vi "MLClassification.vi"(9 "with labels?":bool, 10 "Frame data":string[](array[string]), 11 "model file (JSON)":path) -> (0 "error out":errorcluster, 1 "metrics":T1, 2 "predicted result":i32[][](graph), 3 "feature trend":dbl[][](graph), 5 "Detected hand sign":i32)   [LabVIEW 2017, in "MachineLearning.lvlib"]
doc: "Demonstrates how to deploy a trained classification model to classify test data."
uses:
  MachineLearning.lvlib
  TypeDefs/Label Setting.ctl
  <vilib>/addons/AML/Common/Classes/AML Analytics Model.lvclass/AML Analytics Model.ctl
  <vilib>/addons/AML/Common/Classes/aml_Read Feature Manipulation Model Type.vi
  <vilib>/addons/AML/Data/Load Testing Data (2D Array).vi
  <vilib>/addons/AML/Analytics and Machine Learning.lvlib
  <vilib>/addons/AML/Common/Classes/AML Analytics Model.lvclass
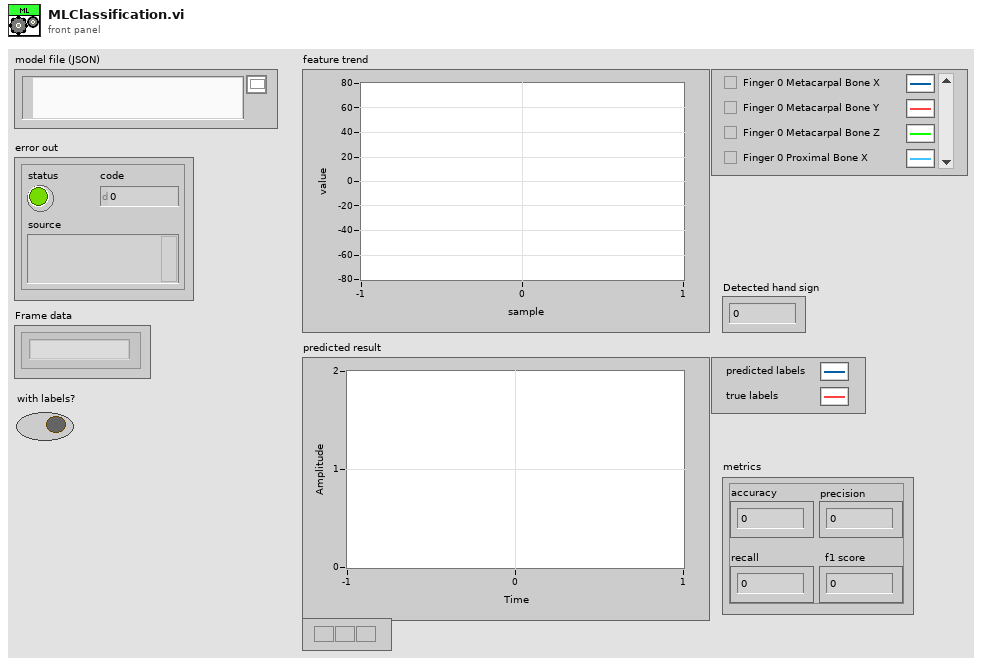
[diagram p1: front panel]
types:
  T1 = cluster{"accuracy":dbl, "precision":dbl, "recall":dbl, "f1 score":dbl}
  T2 = typedef "MachineLearning.lvlib/Label Setting.ctl" = cluster{"with label column?":bool, "label column index":i32}
  T3 = typedef "Analytics and Machine Learning.lvlib/aml_Feature Manipulation Model Type.ctl" = enum16{"None", "Normalize", "Fisher", "PCA", "KPCA"}
  T4 = typedef "Analytics and Machine Learning.lvlib/aml_Model Metrics.ctl" = cluster{"accuracy":dbl, "precision":dbl, "recall":dbl, "f1 score":dbl}
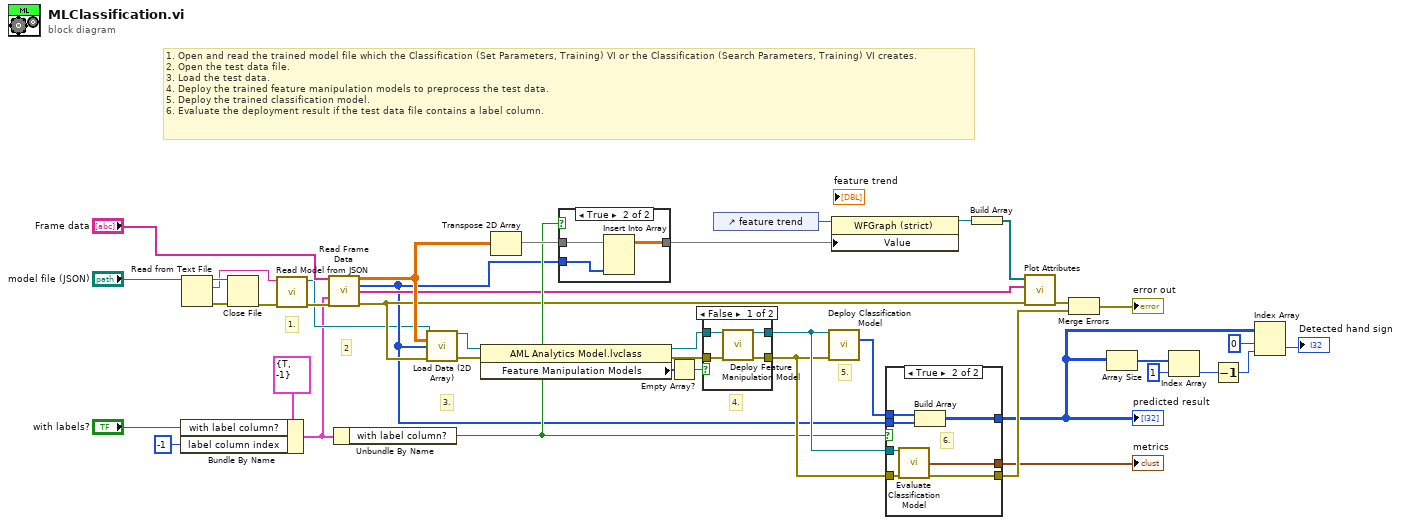
[diagram p0: block diagram]
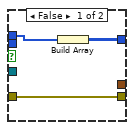
[diagram p2: hidden frame]
diagram:
  # "2"
  # "5."
  # "4."
  # "3."
  # "1."
  # "1. Open and read the trained model file which the Classification (Set Parameters, Training) VI or the Classification (Search Parameters, Training) VI creates.\n2. Open the test data file.\n3. Load the test data.\n4. Deploy the trained feature manipulation models to preprocess the test data.\n5. Deploy the trained classification model.\n6. Evaluate the deployment result if the test data file contains a label column."
  n1 = Bundle By Name(cluster=T2 {"with label column?"=TRUE, "label column index"=-1} ("Label setting"), "with label column?"="with labels?", "label column index"=-1) -> (w1:T2)
  n2 = Read from Text File(file (use dialog)="model file (JSON)") -> (refnum out=w40:refnum<file>, text=w15:string, error out=w41:errorcluster)  [unwired: 3 in, 1 out]
  n3 = Close File(refnum=w40, error in=w41) -> (error out=w14:errorcluster)  [unwired: 1 out]
  n4 = call "Read Model from JSON.vi"("error in (no error)"=w14, "JSON string"=w15) -> ("error out"=w13:errorcluster, "model out"=w12:refnum<class "AML Analytics Model.lvclass">)  [unwired: 6 in, 2 out]
  n5 = call "Read Frame Data.vi"("Frame data"="Frame data", "Label setting"=w1, "error in (no error)"=w13) -> ("data"=w20:dbl[][], "Hand sign"=w17:i32[], "feature names"=w19:string[], "error out"=w18:errorcluster)  [unwired: 9 in]
  n6 = Unbundle By Name(w1) -> ("with label column?"=w23:bool)
  n7 = call-poly <vilib>:"Load Data (2D Array).vi"("model in"=w12, "data"=w20, "data labels"=w17, "error in (no error)"=w18) -> ("model out"=w39:refnum<class "AML Analytics Model.lvclass">, "error out"=w34:errorcluster)  [unwired: 10 in]
  n8 = property class="AML Analytics Model.lvclass"(reference=w39, error in=w34) -> (reference out=w38:refnum<class "AML Analytics Model.lvclass">, error out=w35:errorcluster, "Feature Manipulation Models"=w37:T3[])
  n9 = Transpose 2D Array(2D array=w20) -> (transposed array=w27:dbl[][])
  n10 = case shown="True" w23 {
    tunnel: w27 -> [w43 w46]
    tunnel: w17 -> [_ w45]
    tunnel: [w43 w44] -> w26
    frame False {
    }
    frame True {
      n11 = Insert Into Array(array=w46, new element=w45) -> (w44:dbl[][])  [unwired: 2 in]
    }
  }
  n12 = Empty Array?(array=w37) -> (empty?=w36:bool)
  n13 = case shown="False" w36 {
    tunnel: [w50 w51] -> w33
    tunnel: [w49 w52] -> w32
    tunnel: w38 -> [w48 w51]
    tunnel: w35 -> [w47 w52]
    frame False {
      n14 = call <vilib>:"Deploy Feature Manipulation Model.vi"("model in"=w48, "error in (no error)"=w47) -> ("model out"=w50:refnum<class "AML Analytics Model.lvclass">, "error out"=w49:errorcluster)  [unwired: 11 in, 1 out]
    }
    frame True {
    }
  }
  n15 = control-ref of="feature trend"() -> (w24:refnum<vi>)
  n16 = call <vilib>:"Deploy Classification Model.vi"("model in"=w33, "error in (no error)"=w32) -> ("predicted labels"=w30:i32[])  [unwired: 10 in, 3 out]
  n17 = property class="WFGraph (strict)"(reference=w24, "Value"=w26) -> (reference out=w28:refnum<vi>)  [unwired: 1 in, 1 out]
  n18 = case shown="True" w23 {
    tunnel: w33 -> [_ w62]
    tunnel: w32 -> [w53 w61]
    tunnel: [w53 w60] -> w31
    tunnel: w30 -> [w55 w59]
    tunnel: [w54 w58] -> w6
    tunnel: [_ w57] -> w29
    tunnel: w17 -> [_ w56]
    frame False {
      n19 = Build Array(w55) -> (w54:i32[][])
    }
    frame True {
      # "6."
      n20 = call <vilib>:"Evaluate Classification Model.vi"("model in"=w62, "error in (no error)"=w61) -> ("metrics"=w57:T4, "error out"=w60:errorcluster)  [unwired: 10 in, 2 out]
      n21 = Build Array(w59, w56) -> (w58:i32[][])
    }
  }
  "predicted result" <- w6
  "metrics" <- w29
  n22 = Build Array(w28) -> (w21:refnum<vi>[])
  n23 = call "Plot Attributes.vi"("error in (no error)"=w18, "feature names"=w19, "appended array"=w21) -> ("error in (no error)"=w22:errorcluster)  [unwired: 8 in]
  n24 = Merge Errors(w22, w31) -> (→"error out":errorcluster)
  n25 = Array Size(array=w6) -> (size(s)=w10:i32[])
  n26 = Index Array(array=w10, index=1) -> (element=w8:i32)
  n27 = Decrement(x=w8) -> (x-1=w7:i32)
  n28 = Index Array(array=w6, index (row)=0, index (col)=w7) -> (element=→"Detected hand sign":i32)
